vi "fgt init.vi"(8 "error in (no error)":errorcluster) -> (0 "error out":errorcluster)   [LabVIEW 2020, in "fgt_SDK.lvlib"]
doc: "Initialize or reinitialize (if already opened) Fluigent SDK instance. All detected Fluigent instruments (MFCS, MFCS-EZ, FRP, LineUP, IPS) are initialized.\nThis function is optional, directly calling a function will automatically creates the instance."
uses:
  fgt_SDK.lvlib
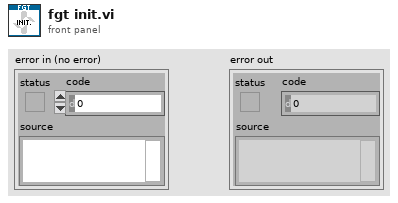
[diagram p1: front panel]
types:
  T1 = typedef "fgt_SDK.lvlib/fgt_STATUS_INFO.ctl" = cluster{"InstrType":T2, "instrSN":u16, "errorCode":u8, "infoCode":u8, "detail":string}
  T2 = typedef "fgt_SDK.lvlib/fgt_INSTRUMENT_TYPE.ctl" = enum32{"None", "MFCS", "MFCS_EZ", "FRP", "LineUP", "IPS"}
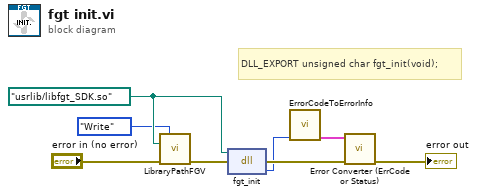
[diagram p0: block diagram]
diagram:
  w2 = path "/usrlib/libfgt_SDK.so"
  # "DLL_EXPORT unsigned char fgt_init(void);"
  n1 = call "LibraryPathFGV.vi"("Action"=enum16{"Read", "Write"}."Write", "Path In"=w2, "error in (no error)"="error in (no error)") -> ("error out"=w3:errorcluster)  [unwired: 11 in, 1 out]
  n2 = dll-call lib="C:/Workspace/fgt-SDK/LabVIEW/dlls/fgt_SDK_*.*" fn="fgt_init"(path in=w2, error in=w3) -> (error out=w8:errorcluster, "return type"=w6:u8)  [unwired: 1 in, 1 out]
  n3 = call "ErrorCodeToErrorInfo.vi"("return type"=w6) -> ("StatusInfo"=w5:T1)  [unwired: 10 in]
  n4 = call "Error Converter (ErrCode or Status).vi"("error in (no error)"=w8, "StatusInfo"=w5) -> ("error out"=→"error out":errorcluster)  [unwired: 9 in]
